vi "UTIL_Check for Equality with Percentage.vi"(8 "error in":errorcluster, 9 "percentage (of Target)":dbl=0.1 format="%.6f", 10 "Number to Check":dbl format="%.9f", 11 "Target Number":dbl format="%.9f") -> (0 "error out":errorcluster, 1 "Target < Check?":bool, 2 "Target > Check?":bool, 3 "equal (within percentage)":bool, 4 "measured percentage":dbl format="%.6f")   [LabVIEW 2010]
doc: "<b>Check two floating point numbers for equality. </b>\n\nEquality is defined as: The \"Number to Check\" is within the specified percentage of the \"Target Number\".\nThe \"percentage\" is relative to the \"Target Number\", not the larger of the two.\n\nModified from: NI_MAPro.liblib:ma_Check for Equality with Precision.vi\n\nCopyright 2010 Michael Ashe, Imaginatics\n(michael.ashe@imaginatics.net)"
panel:
  # "C:\\Program Files\\National Instruments\\LabVIEW 2010\\vi.lib\\measure\\mamon.llb\\ma_Check for Equality with Precision.vi"
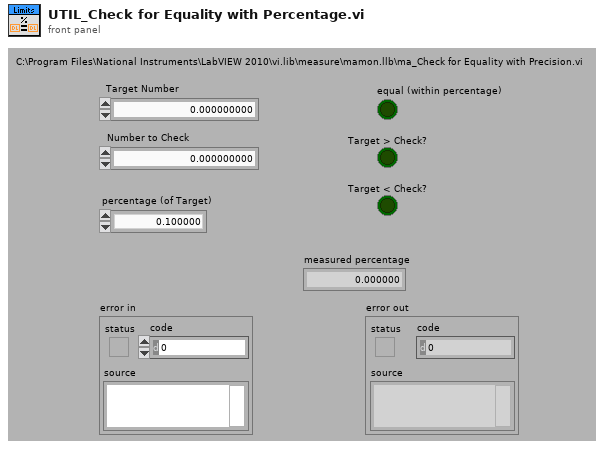
[diagram p1: front panel]
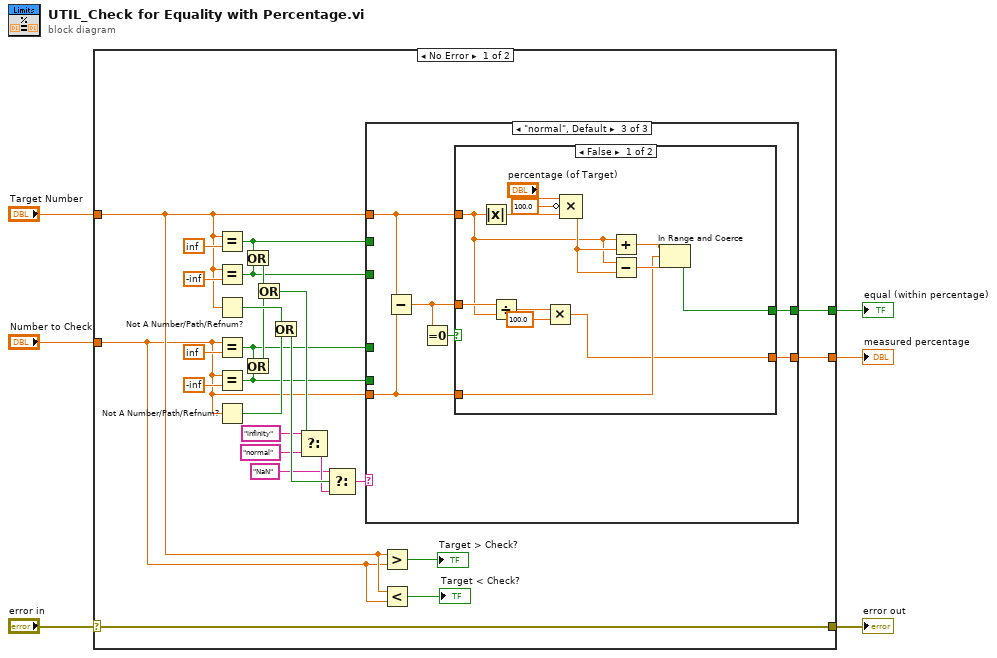
[diagram p0: block diagram]
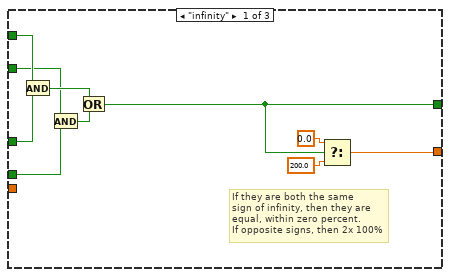
[diagram p2: hidden frame]
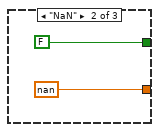
[diagram p3: hidden frame]
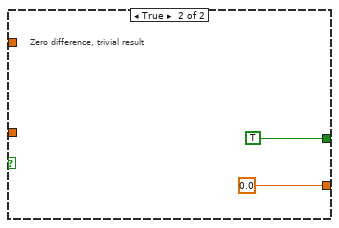
[diagram p4: hidden frame]
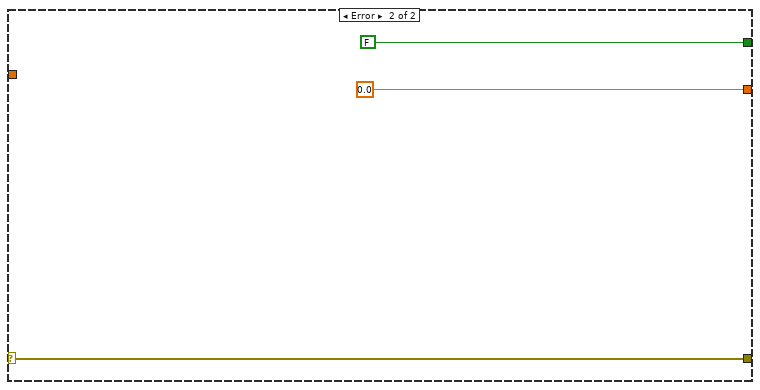
[diagram p5: hidden frame]
diagram:
  n1 = case shown="No Error" "error in" {
    selector: "error in" -> [w7 w68]
    tunnel: [w13 FALSE] -> w6
    tunnel: [w12 0.0 ("measured percentage")] -> w5
    tunnel: "Target Number" -> [w11 _]
    tunnel: "Number to Check" -> [w10 _]
    tunnel: [w7 w68] -> w1
    frame No Error {
      n2 = Equal?(x=w11, y=inf) -> (x = y?=w16:bool)
      n3 = Equal?(x=w11, y=-inf) -> (x = y?=w17:bool)
      n4 = Not A Number/Path/Refnum?(number/path/refnum=w11) -> (NaN/Path/Refnum?=w28:bool)
      n5 = Equal?(x=w10, y=inf) -> (x = y?=w15:bool)
      n6 = Equal?(x=w10, y=-inf) -> (x = y?=w14:bool)
      n7 = Not A Number/Path/Refnum?(number/path/refnum=w10) -> (NaN/Path/Refnum?=w27:bool)
      n8 = Or(x=w16, y=w17) -> (x .or. y?=w26:bool)
      n9 = Or(x=w15, y=w14) -> (x .or. y?=w25:bool)
      n10 = Or(x=w26, y=w25) -> (x .or. y?=w24:bool)
      n11 = Or(x=w28, y=w27) -> (x .or. y?=w23:bool)
      n12 = Select(t="infinity", s=w24, f="normal") -> (s? t:f=w22:string)
      n13 = Select(t="NaN", s=w23, f=w22) -> (s? t:f=w18:string)
      n14 = case shown="\"normal\", Default" w18 {
        tunnel: [w35 FALSE w47] -> w13
        tunnel: [w36 nan w46] -> w12
        tunnel: w17 -> [w37 _ _]
        tunnel: w16 -> [w42 _ _]
        tunnel: w15 -> [w41 _ _]
        tunnel: w14 -> [w38 _ _]
        tunnel: w11 -> [_ _ w49]
        tunnel: w10 -> [_ _ w48]
        frame "infinity" {
          # "If they are both the same\nsign of infinity, then they are\nequal, within zero percent.\nIf opposite signs, then 2x 100%"
          n15 = And(x=w42, y=w41) -> (x .and. y?=w40:bool)
          n16 = And(x=w37, y=w38) -> (x .and. y?=w39:bool)
          n17 = Or(x=w40, y=w39) -> (x .or. y?=w35:bool)
          n18 = Select(t=0.0, s=w35, f=200.0) -> (s? t:f=w36:dbl)
        }
        frame "NaN" {
        }
        frame "normal", Default {
          n19 = Subtract(x=w49, y=w48) -> (x-y=w45:dbl)
          n20 = Equal To 0?(x=w45) -> (x = 0?=w50:bool)
          n21 = case shown="False" w50 {
            tunnel: w45 -> [w55 _]
            tunnel: w49 -> [w54 _]
            tunnel: w48 -> [w57 _]
            tunnel: [w56 TRUE] -> w47
            tunnel: [w51 0.0] -> w46
            frame False {
              n22 = Absolute Value(x=w54) -> (abs(x)=w61:dbl)
              n23 = Divide(x=w55, y=w54) -> (x/y=w53:dbl)
              n24 = Multiply(x=w53, y=100.0) -> (x*y=w51:dbl)
              n25 = Compound Arithmetic op=MULTIPLY("percentage (of Target)", invert 100.0 ("value"), w61) -> (w60:dbl)
              n26 = Add(x=w54, y=w60) -> (x+y=w58:dbl)
              n27 = Subtract(x=w54, y=w60) -> (x-y=w59:dbl)
              n28 = In Range and Coerce(upper limit=w58, x=w57, lower limit=w59) -> (In Range?=w56:bool)  [unwired: 1 out]
            }
            frame True {
              # "Zero difference, trivial result"
            }
          }
        }
      }
      n29 = Greater?(x=w11, y=w10) -> (0:→"Target > Check?":bool)
      n30 = Less?(x=w11, y=w10) -> (x < y?=→"Target < Check?":bool)
    }
    frame Error {
    }
  }
  "measured percentage" <- w5
  "equal (within percentage)" <- w6
  "error out" <- w1
